vi "TDS DCPS Set Current.vi"(8 "error in (no error)":errorcluster, 9 "Current":dbl, 10 "Signal InstConfig":string, 11 "Address":string) -> (0 "error out":errorcluster)   [LabVIEW 2025, in "Interface Functions.lvlib"]
uses:
  Interface Functions.lvlib
panel:
  # "DCPS Set Current"
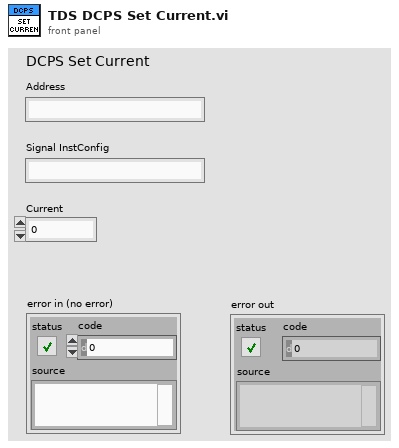
[diagram p1: front panel]
types:
  T1 = typedef "Interface Functions.lvlib/Current Limit Mode--enum.ctl" = enum16{"REGULATE", "TRIP"}
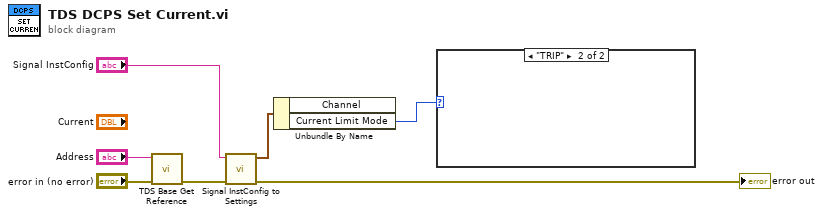
[diagram p0: block diagram]
diagram:
  n1 = call "TDS Base Get Reference.vi"("error in (no error)"="error in (no error)", "Address"="Address") -> ("error out"=w5:errorcluster)  [unwired: 8 in, 1 out]
  n2 = call "Signal InstConfig to Settings.vi"("error in (no error)"=w5, "Signal InstConfig"="Signal InstConfig") -> ("error out"=→"error out":errorcluster, "Settings"=w3:cluster{"Channel":i32, "Current Limit Mode":T1})  [unwired: 8 in]
  n3 = Unbundle By Name(w3) -> ("Current Limit Mode"=w1:T1)  [unwired: 1 out]
  n4 = case shown="\"TRIP\"" w1 {
    frame "REGULATE", Default {
    }
    frame "TRIP" {
    }
  }
